vi "Simple Wait in us.vi"(1 "Wait(us)":u32=100000 format="%.0p") -> ()   [LabVIEW 2024]
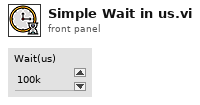
[diagram p1: front panel]
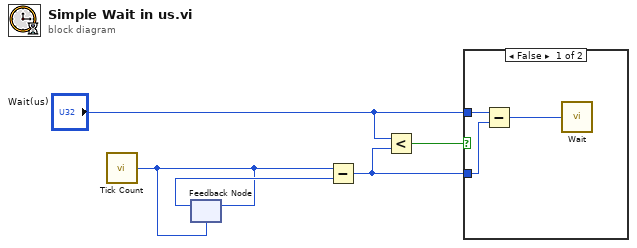
[diagram p0: block diagram]
diagram:
  n1 = call "Tick Count"() -> ("Tick Count(uSec)"=w1:u32)
  n2 = feedback #1(w1) -> (w2:u32)
  n3 = feedback-in #1(w1) -> ()
  n4 = Subtract(x=w1, y=w2) -> (x-y=w5:u32)
  n5 = Less?(x="Wait(us)", y=w5) -> (x < y?=w4:bool)
  n6 = case shown="False" w4 {
    tunnel: "Wait(us)" -> [w8 _]
    tunnel: w5 -> [w7 _]
    frame False {
      n7 = Subtract(x=w8, y=w7) -> (x-y=w6:u32)
      n8 = call "Wait"("Count(uSec)"=w6) -> ()  [unwired: 1 out]
    }
    frame True {
    }
  }
